vi "Convert State For Save.vi"(2 "Container State":T1, 3 "Display State":T2) -> (1 "Display State To Save":variant)   [LabVIEW 2020, in "2D Feather.xctl"]
uses:
  <vilib>/Math Plots/2D Math Plots/2D Feather/2D Feather XCtrl/2D Feather.xctl
  <vilib>/Math Plots/2D Math Plots/2D Feather/2D Feather XCtrl/State.ctl
  <vilib>/Math Plots/2D Math Plots/2D Feather/2D Feather/2D Feather.lvclass
  e:/builds/penguin/labview/branches/2020/dev/dist/vi.lib/Math Plots/2D Math Plots/2D Plot/2D Plot/2D Plot.lvclass
  <vilib>/Math Plots/2D Math Plots/2D Plot/Action String/2DMathPlot Ctrl Act Queue.ctl
  <vilib>/Math Plots/2D Math Plots/2D Plot/Action String/2DMathPlot Ctrl Act Cluster.ctl
  <vilib>/Math Plots/2D Math Plots/2D Plot/Action String/2DMathPlot State Class.ctl
  <vilib>/_xctls/Container State.ctl
  <vilib>/Math Plots/2D Math Plots/2D Plot/2D Plot/2D Plot.lvclass
  <vilib>/_xctls/XControlSupport.lvlib
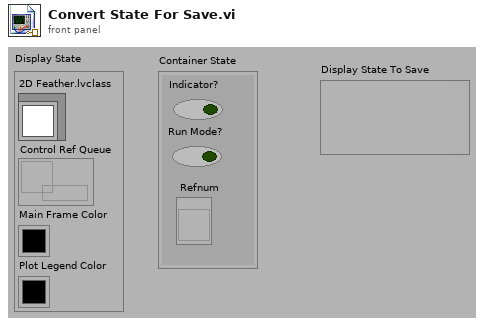
[diagram p1: front panel]
types:
  T1 = typedef "XControlSupport.lvlib/Container State.ctl" = cluster{"Indicator?":bool, "Run Mode?":bool, " Refnum":refnum<vi>}
  T2 = typedef "2D Feather.xctl/State.ctl" = cluster{"2D Feather.lvclass":refnum<class "2D Feather.lvclass">, "Control Ref Queue":T3, "Main Frame Color":u32, "Plot Legend Color":u32}
  T3 = typedef "2DMathPlot Ctrl Act Queue.ctl" = refnum<queue>
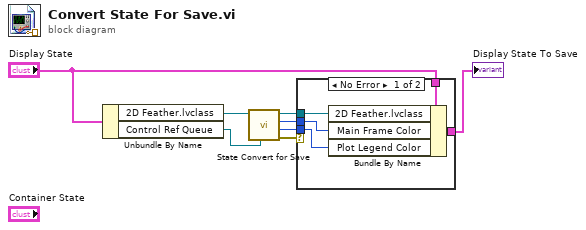
[diagram p0: block diagram]
diagram:
  n1 = Unbundle By Name("Display State") -> ("2D Feather.lvclass"=w6:refnum<class "2D Feather.lvclass">, "Control Ref Queue"=w5:T3)
  n2 = call <vilib>:"State Convert for Save.vi"("Control Ref Queue"=w5, "2D Plot.lvclass"=w6) -> ("error out"=w1:errorcluster, "Plot Legend Color"=w2:u32, "Main Frame Color"=w3:u32, "2D Plot.lvclass out"=w4:refnum<class "2D Feather.lvclass">)  [unwired: 2 in, 4 out]
  n3 = case shown="No Error" w1 {
    tunnel: "Display State" -> [w13 w14]
    tunnel: [w12 w14] -> w7
    tunnel: w4 -> [w11 _]
    tunnel: w3 -> [w10 _]
    tunnel: w2 -> [w9 _]
    frame No Error {
      n4 = Bundle By Name(cluster=w13, "2D Feather.lvclass"=w11, "Main Frame Color"=w10, "Plot Legend Color"=w9) -> (w12:T2)
    }
    frame Error {
    }
  }
  "Display State To Save" <- w7
